vi "Close Measurement.vi"(8 "error in":errorcluster, 11 "gRPCid in":u64) -> (0 "error out":errorcluster)   [LabVIEW 2021, in "Measurement Client Template.lvlib"]
uses:
  Measurement Client Template.lvlib
  <vilib>/gRPC/Generated APIs/ni/measurementlink/measurement/v2/Measurement Service Client/Measurement Service Client.lvlib
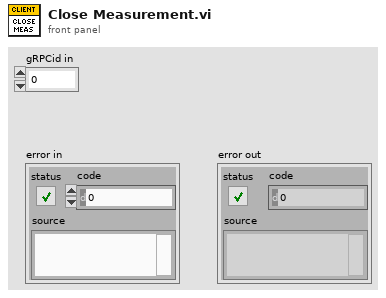
[diagram p1: front panel]
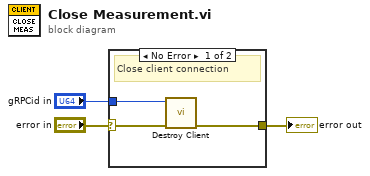
[diagram p0: block diagram]
diagram:
  n1 = case shown="No Error" "error in" {
    selector: "error in" -> [w4 w7]
    tunnel: "gRPCid in" -> [w6 _]
    tunnel: [w5 w7] -> w2
    frame No Error {
      # "Close client connection"
      n2 = call <vilib>:"Destroy Client.vi"("error in"=w4, "gRPC ID"=w6) -> ("error out"=w5:errorcluster)  [unwired: 9 in]
    }
    frame Error {
      # "Pass"
    }
  }
  "error out" <- w2
